vi "Strip Path To Token.vi"(8 "Error In":errorcluster, 10 "Token (Regex)":string=".exe", 11 "Path":path) -> (0 "Error Out":errorcluster, 1 "Found Token?":bool, 3 "Stripped Path":path)   [LabVIEW 2011, in "LMH-Toolbox.lvlib" / "LMH-Common.lvlib"]
doc: "Given a path and a Token (regular expression) this VI returns the file path stripped to the token.\n\nFor example the following token will strip the path to the <LabVIEW> directory:\n\nToken: LabVIEW [0-9]+.?[0-9]? \nPath: C:\\Program Files (x86)\\National Instruments\\LabVIEW 2011\\vi.lib\\LabVIEW Hacker\\LVH Toolbox\\Test.vi\n\nReturns C:\\Program Files (x86)\\National Instruments\\LabVIEW 2011"
uses:
  LMH-Common.lvlib
  <vilib>/regexp/Match Regular Expression.xnode
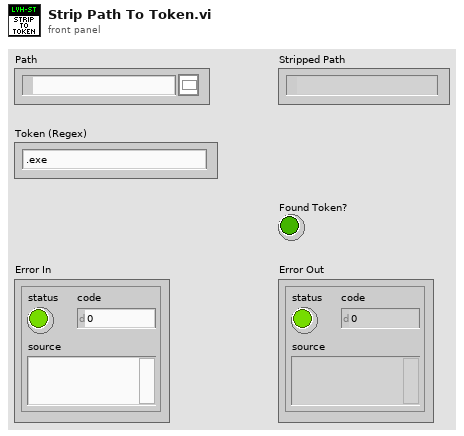
[diagram p1: front panel]
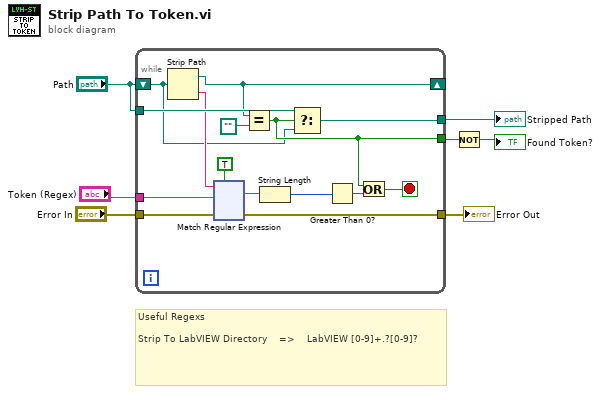
[diagram p0: block diagram]
diagram:
  # "Useful Regexs\n\nStrip To LabVIEW Directory    =>    LabVIEW [0-9]+.?[0-9]?"
  n1 = while {
    shift-right: [w18] -> _
    shift-left: "Path" -> [w10]
    tunnel: "Path" -> [w19]
    tunnel: [w17] -> w6
    tunnel: [w16] -> w5
    tunnel: "Token (Regex)" -> [w14]
    tunnel: "Error In" -> [w9]
    tunnel: [w8] -> w1
    stop <- w20 stop-if-true
    n2 = Strip Path(path=w10) -> (stripped path=w18:path, name=w15:string)
    n3 = xnode "Match Regular Expression"("input string"=w15, "regular expression"=w14, "error in"=w9, "ignore case? (F)"=TRUE) -> ("whole match"=w11:string, "error out"=w8:errorcluster)  [unwired: 2 in, 3 out]
    n4 = Equal?(x=w18, y=path "") -> (x = y?=w16:bool)
    n5 = String Length(string=w11) -> (length=w12:i32)
    n6 = Select(t=w19, s=w16, f=w10) -> (s? t:f=w17:path)
    n7 = Greater Than 0?(x=w12) -> (x > 0?=w21:bool)
    n8 = Or(x=w16, y=w21) -> (x .or. y?=w20:bool)
  }
  "Stripped Path" <- w6
  "Error Out" <- w1
  n9 = Not(x=w5) -> (.not. x?=→"Found Token?":bool)
